vi "test_Check String Comparison_first expected string is found if multiples.vi"(8 "error in (no error)":errorcluster, 11 "TestCase in":refnum<class "Instrument Addon Unit Tests.lvclass">) -> (0 "error out":errorcluster, 3 "TestCase out":refnum<class "Instrument Addon Unit Tests.lvclass">)   [LabVIEW 2020, in "Instrument Addon Unit Tests.lvclass"]
uses:
  Instrument Addon Unit Tests.lvclass
  <vilib>/addons/_JKI Toolkits/VI Tester/TestCase.llb/TestCase.lvclass
  Addon/Addon Engine/Instrument Addon Engine.lvlib
  C:/Program Files (x86)/National Instruments/LabVIEW 2020/vi.lib/addons/_JKI Toolkits/VI Tester/TestCase.llb/TestCase.lvclass
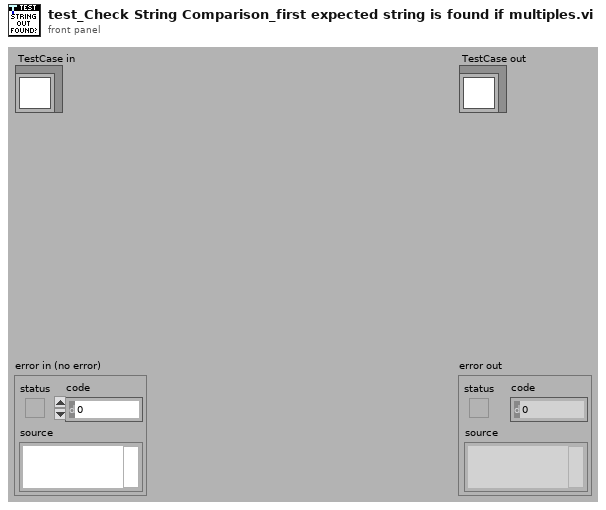
[diagram p1: front panel]
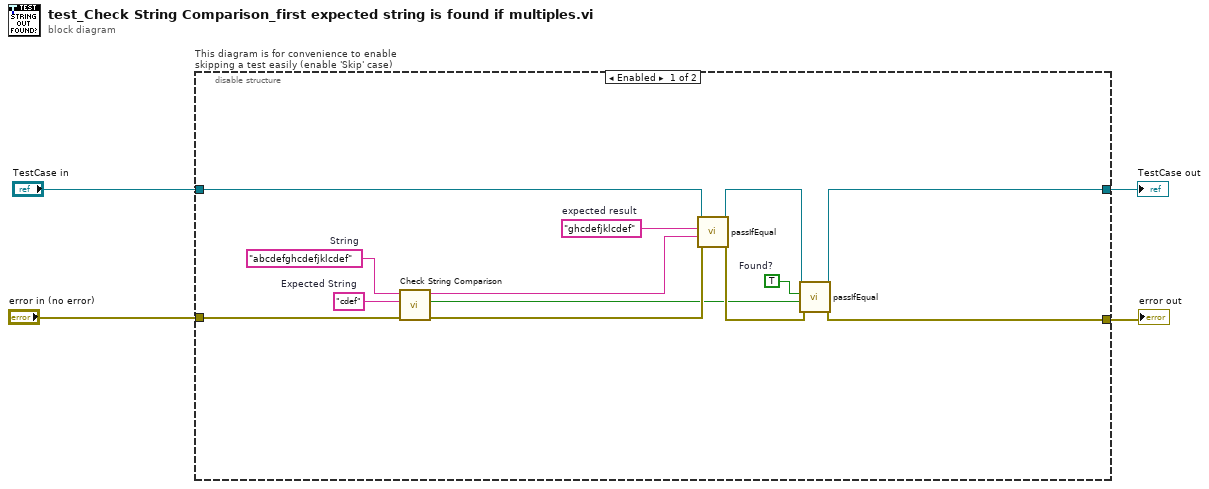
[diagram p0: block diagram]
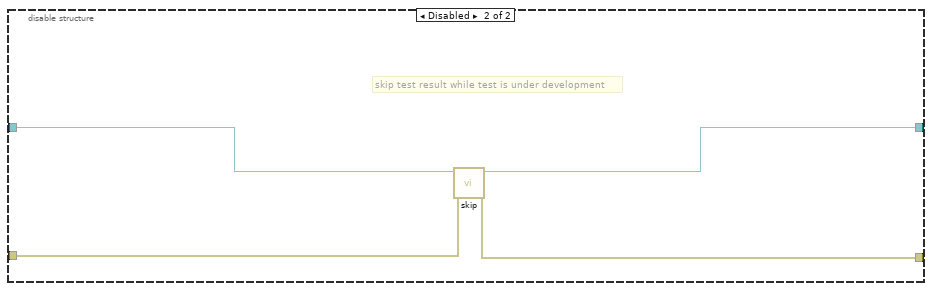
[diagram p2: hidden frame]
diagram:
  n1 = disable-structure "This diagram is for convenience to enable skipping a test easily (enable 'Skip' case)" shown="Enabled" {
    disable-tunnel: "TestCase in" -> [w16 w21]
    disable-tunnel: [w10 w19] -> w1
    disable-tunnel: [w7 w20] -> w3
    disable-tunnel: "error in (no error)" -> [w15 w18]
    frame Enabled {
      w5 = TRUE  # Found?
      w11 = "cdef"  # Expected String
      w12 = "abcdefghcdefjklcdef"  # String
      w17 = "ghcdefjklcdef"  # expected result
      n2 = call "Check String Comparison.vi"("error in (no error)"=w15, "Expected String"=w11, "String"=w12) -> ("error out"=w14:errorcluster, "Found?"=w6:bool, "string out"=w13:string)  [unwired: 6 in]
      n3 = call-dynamic "passIfEqual.vi"("error in (no error)"=w14, "y"=w13, "x"=w17, "TestCase in"=w16) -> ("error out"=w8:errorcluster, "TestCase out"=w9:refnum<class "Instrument Addon Unit Tests.lvclass">)  [unwired: 6 in]
      n4 = call-dynamic "passIfEqual.vi"("error in (no error)"=w8, "y"=w6, "x"=w5, "TestCase in"=w9) -> ("error out"=w7:errorcluster, "TestCase out"=w10:refnum<class "Instrument Addon Unit Tests.lvclass">)  [unwired: 6 in]
    }
    frame Disabled {
      # "skip test result while test is under development"
      n5 = call <vilib>:"skip.vi"("error in (no error)"=w18, "TestCase in"=w21) -> ("error out"=w20:errorcluster, "TestCase out"=w19:refnum<class "Instrument Addon Unit Tests.lvclass">)  [unwired: 8 in]
    }
  }
  "error out" <- w3
  "TestCase out" <- w1
